vi "Read Channel Names.vi"(8 "error in (no error)":errorcluster, 11 "Telescope in":refnum<class "Telescope.lvclass">) -> (0 "error out":errorcluster, 2 "Channel Names":string[](array[string])=["Telescope RA", "Telescope DEC", "Telescope Moving?", "Telescope Status"], 3 "Telescope out":refnum<class "Telescope.lvclass">)   [LabVIEW 2022 SP3, in "Telescope.lvclass"]
uses:
  Telescope.lvclass
  Telescope.lvclass/Telescope.ctl
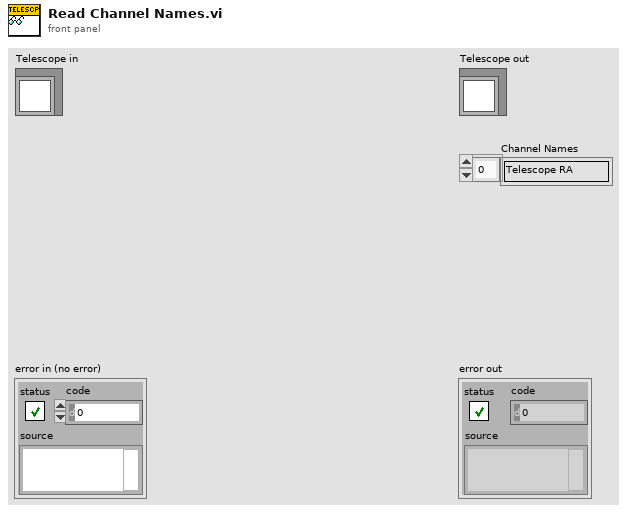
[diagram p1: front panel]
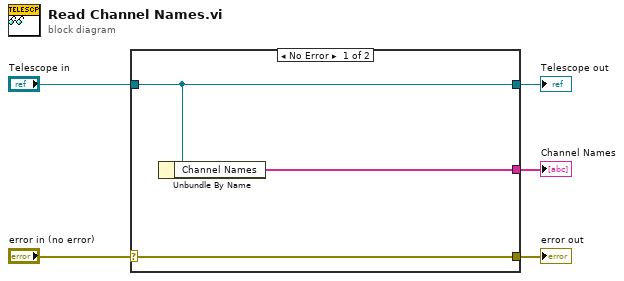
[diagram p0: block diagram]
diagram:
  n1 = case shown="No Error" "error in (no error)" {
    selector: "error in (no error)" -> [w8 w9]
    tunnel: [w8 w9] -> w4
    tunnel: [w7 w10] -> w2
    tunnel: "Telescope in" -> [w7 w10]
    tunnel: [w6 _] -> w1
    frame No Error {
      n2 = Unbundle By Name(w7) -> ("Channel Names"=w6:string[])
    }
    frame Error {
    }
  }
  "error out" <- w4
  "Telescope out" <- w2
  "Channel Names" <- w1
